vi "BeforeStart.vi"(8 "error in (no error)":errorcluster) -> (0 "error out":errorcluster, 1 "x = y?":bool, 3 "ref path":path)   [LabVIEW 2017]
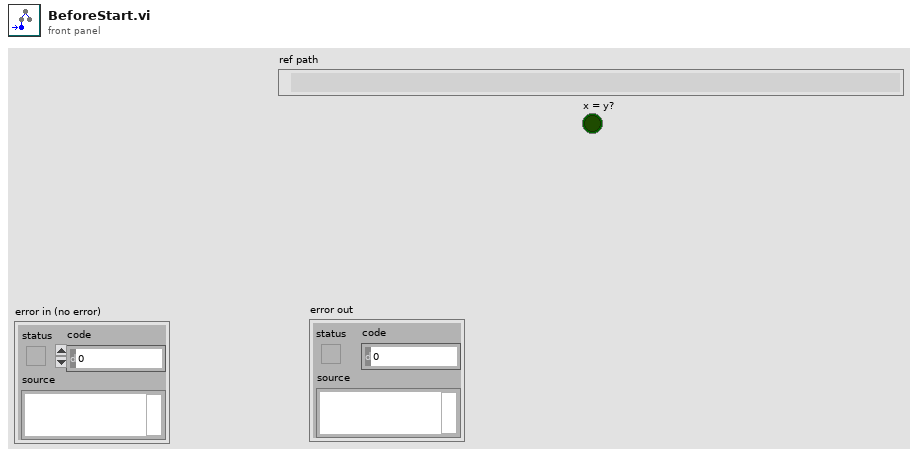
[diagram p1: front panel]
types:
  T1 = enum32{"invalid app kind", "Development System", "Run Time System", "Student Edition", "Embedded LabVIEW", "Evaluation", "Custom"}
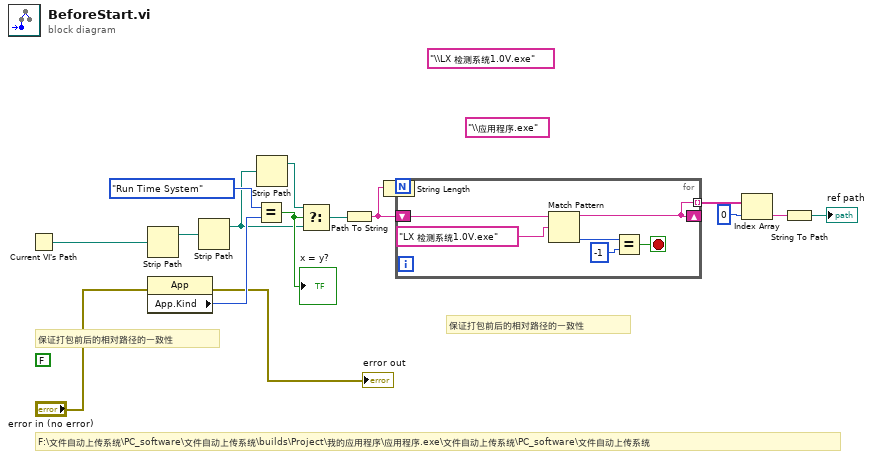
[diagram p0: block diagram]
diagram:
  (unwired) "\\LX 检测系统1.0V.exe" ("子字符串(\"\")")
  (unwired) "\\应用程序.exe" ("子字符串(\"\")")
  (unwired) FALSE ("exit app?")
  # "保证打包前后的相对路径的一致性"
  # "F:\\文件自动上传系统\\PC_software\\文件自动上传系统\\builds\\Project\\我的应用程序\\应用程序.exe\\文件自动上传系统\\PC_software\\文件自动上传系统"
  # "保证打包前后的相对路径的一致性"
  n1 = Current VI's Path() -> (path=w13:path)
  n2 = Strip Path(path=w13) -> (stripped path=w12:path)  [unwired: 1 out]
  n3 = property class="App"(error in="error in (no error)") -> (error out=→"error out":errorcluster, "App.Kind"=w15:T1)  [unwired: 1 in, 1 out]
  n4 = Strip Path(path=w12) -> (stripped path=w11:path)  [unwired: 1 out]
  n5 = Equal?(x=T1."Run Time System" ("Application:Kind"), y=w15) -> (x = y?=w14:bool)
  "x = y?" <- w14
  n6 = Strip Path(path=w11) -> (stripped path=w10:path)  [unwired: 1 out]
  n7 = Select(t=w10, s=w14, f=w11) -> (s? t:f=w9:path)
  n8 = Path To String(path=w9) -> (string=w5:string)
  n9 = String Length(string=w5) -> (length=w8:i32)
  n10 = for {
    N: w8 -> [_]
    shift-right: [w19] -> _
    shift-left: w5 -> [w22]
    tunnel: [w19] -> w7 mode=indexing
    stop <- w20 stop-if-true
    n11 = Match Pattern(string=w22, regular expression="LX 检测系统1.0V.exe" ("子字符串(\"\")")) -> (before substring=w19:string, offset past match=w17:i32)  [unwired: 1 in, 2 out]
    n12 = Equal?(x=w17, y=-1) -> (x = y?=w20:bool)
  }
  n13 = Index Array(array=w7, index=0 ("索引")) -> (element=w3:string)
  n14 = String To Path(string=w3) -> (path=→"ref path":path)
